vi "Get Common Panel Controls Values.vi"(0 "Schedule Block in":refnum<class "Schedule Block.lvclass">, 11 "error in (no error)":errorcluster) -> (3 "Script Path":path, 4 "Schedule Block out":refnum<class "Schedule Block.lvclass">, 6 "Script Name":string, 8 "Common Parameters":string[][](array[string]), 10 "Number of repetitions":u16, 14 "FPGA Name":string, 15 "error out":errorcluster)   [LabVIEW 2020, in "TALOS.lvlib" / "Run Utilities.lvlib" / "Schedule Block.lvclass"]
uses:
  Schedule Block.lvclass
  Schedule Block.lvclass/Schedule Block.ctl
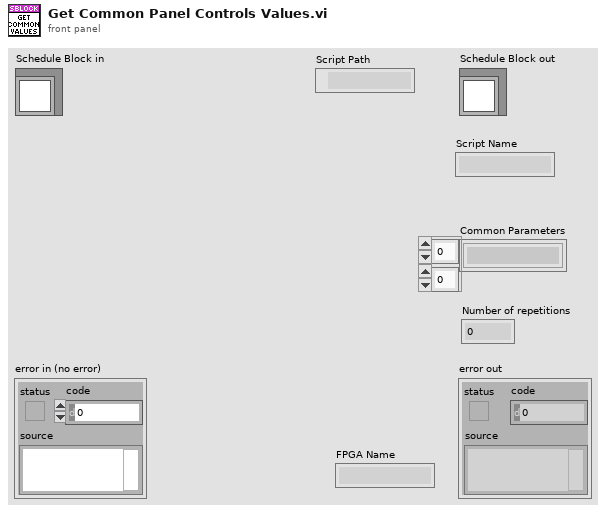
[diagram p1: front panel]
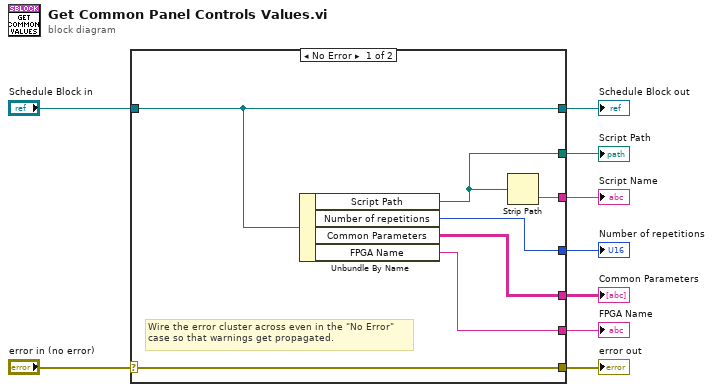
[diagram p0: block diagram]
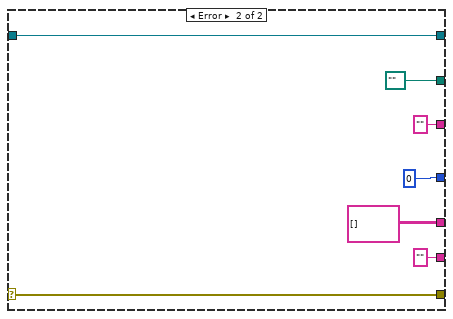
[diagram p2: hidden frame]
diagram:
  n1 = case shown="No Error" "error in (no error)" {
    selector: "error in (no error)" -> [w16 w23]
    tunnel: [w16 w23] -> w8
    tunnel: [w15 w22] -> w6
    tunnel: "Schedule Block in" -> [w15 w22]
    tunnel: [w12 path "" ("Script Path")] -> w5
    tunnel: [w14 u16 0 ("Number of repetitions")] -> w4
    tunnel: [w13 string[][] [] ("Common Parameters")] -> w3
    tunnel: [w10 ""] -> w2
    tunnel: [w11 "" ("name")] -> w1
    frame No Error {
      # "Wire the error cluster across even in the \"No Error\"\ncase so that warnings get propagated."
      n2 = Unbundle By Name(w15) -> ("Script Path"=w12:path, "Number of repetitions"=w14:u16, "Common Parameters"=w13:string[][], "FPGA Name"=w10:string)
      n3 = Strip Path(path=w12) -> (name=w11:string)  [unwired: 1 out]
    }
    frame Error {
    }
  }
  "error out" <- w8
  "Schedule Block out" <- w6
  "Script Path" <- w5
  "Number of repetitions" <- w4
  "Common Parameters" <- w3
  "FPGA Name" <- w2
  "Script Name" <- w1
